vi "Set Control On.vi"(8 "error in (no error)":errorcluster, 11 "VISA resource name":refnum<visa-resource-name>="COM3") -> (0 "error out":errorcluster, 3 "VISA resource name out":refnum<visa-resource-name>)   [LabVIEW 2017]
doc: "This changes the temperature setpoint. If you want to query the setpoint after this, make sure there is a 0.2 s delay (according to manual)."
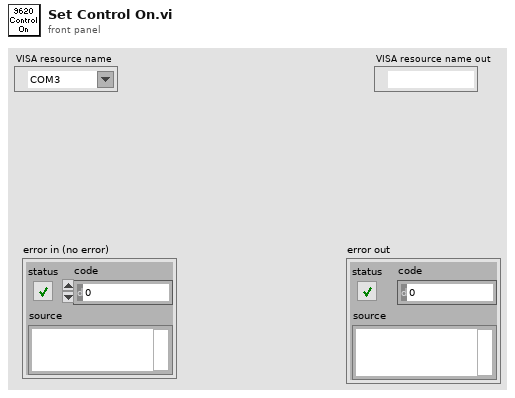
[diagram p1: front panel]
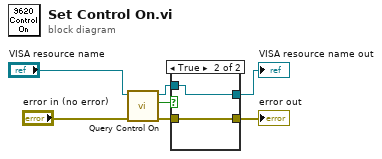
[diagram p0: block diagram]
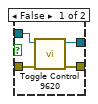
[diagram p2: hidden frame]
diagram:
  n1 = call "Query Control On.vi"("error in (no error)"="error in (no error)", "VISA resource name"="VISA resource name") -> ("error out"=w3:errorcluster, "Control on?"=w5:bool, "VISA resource name out"=w4:refnum<visa-resource-name>)  [unwired: 7 in]
  n2 = case shown="True" w5 {
    tunnel: w4 -> [w11 w13]
    tunnel: w3 -> [w10 w12]
    tunnel: [w9 w13] -> w2
    tunnel: [w8 w12] -> w1
    frame False {
      n3 = call "Toggle Control 9620.vi"("error in (no error)"=w10, "VISA resource name"=w11) -> ("error out"=w8:errorcluster, "VISA resource name out"=w9:refnum<visa-resource-name>)  [unwired: 8 in]
    }
    frame True {
    }
  }
  "VISA resource name out" <- w2
  "error out" <- w1
